vi "_readBoolean.vi"(8 "error in (no error)":errorcluster, 11 "tJSONParser in":refnum<class "tJSONParser.lvclass">) -> (0 "error out":errorcluster, 2 "tBSONBoolean out":refnum<class "tBSONBoolean.lvclass">, 3 "tJSONParser out":refnum<class "tJSONParser.lvclass">)   [LabVIEW 2013, in "JSON.lvlib" / "tJSONParser.lvclass"]
doc: "Reads and validates a boolean value from a string : value pair."
uses:
  tJSONParser.lvclass
  BSON/BSONElements/tBSONBoolean/tBSONBoolean.lvclass
  _error.ctl
  BSON/BSONElements/tBSONBoolean/setValue.vi
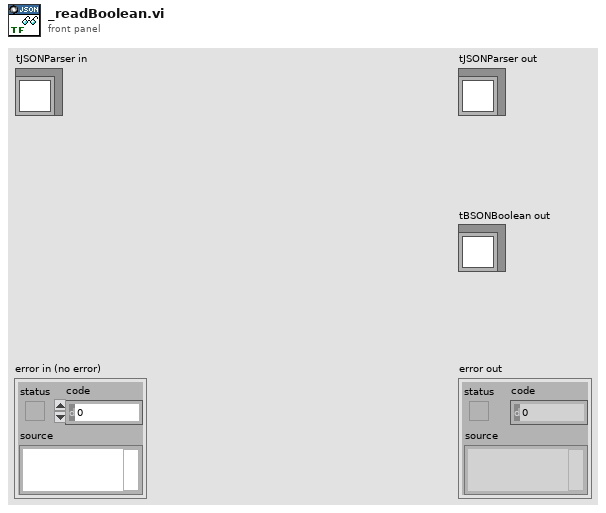
[diagram p1: front panel]
types:
  T1 = typedef "JSON.lvlib/tJSONParser.lvclass/_error.ctl" = enum16{"Missing Object Open", "Missing Pair Separator", "Missing Object End Or Separator", "Missing Pair String", "Unexpected Token", "Missing Array End Or Separator", "Invalid Escape Sequence", "Unexpected End Of File", "Invalid Unicode", "Unexpected End Of Line", "Invalid Numerical Constant"}
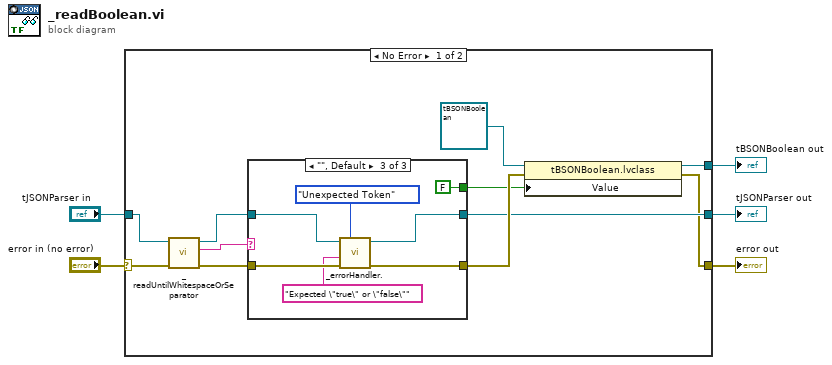
[diagram p0: block diagram]
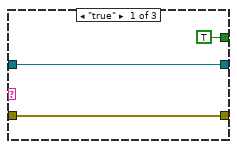
[diagram p2: hidden frame]
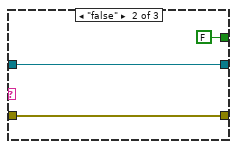
[diagram p3: hidden frame]
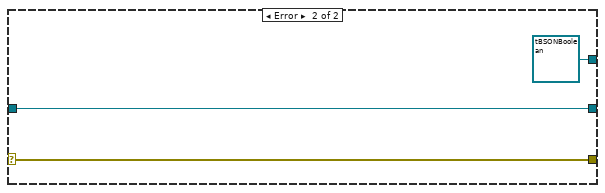
[diagram p4: hidden frame]
diagram:
  n1 = case shown="No Error" "error in (no error)" {
    selector: "error in (no error)" -> [w16 w32]
    tunnel: [w11 w32] -> w4
    tunnel: [w12 w31] -> w2
    tunnel: "tJSONParser in" -> [w8 w31]
    tunnel: [w10 refnum<class "tBSONBoolean.lvclass"> refnum ("lvMongoDriver.lvlib:BSON.lvlib:tBSONBoolean.lvclass")] -> w1
    frame No Error {
      n2 = call "_readUntilWhitespaceOrSeparator.vi"("error in (no error)"=w16, "tJSONParser in"=w8) -> ("error out"=w6:errorcluster, "String Out"=w7:string, "tJSONParser out"=w15:refnum<class "tJSONParser.lvclass">)  [unwired: 7 in]
      n3 = case shown="\"\", Default" w7 {
        tunnel: w6 -> [w18 w22 w29]
        tunnel: w15 -> [w19 w21 w28]
        tunnel: [w19 w21 w25] -> w12
        tunnel: [w18 w22 w24] -> w13
        tunnel: [TRUE FALSE FALSE] -> w9
        frame "true" {
        }
        frame "false" {
        }
        frame "", Default {
          n4 = call "_errorHandler..vi"("error in (no error)"=w29, "Additional Text"="Expected \"true\" or \"false\"", "Error Type"=_error."Unexpected Token", "JSON Parser In"=w28) -> ("error out"=w24:errorcluster, "JSON Parser Out"=w25:refnum<class "tJSONParser.lvclass">)  [unwired: 6 in]
        }
      }
      n5 = property class="tBSONBoolean.lvclass"(reference=refnum<class "tBSONBoolean.lvclass"> refnum ("lvMongoDriver.lvlib:BSON.lvlib:tBSONBoolean.lvclass"), error in=w13, "Value"=w9) -> (reference out=w10:refnum<class "tBSONBoolean.lvclass">, error out=w11:errorcluster)
    }
    frame Error {
    }
  }
  "error out" <- w4
  "tJSONParser out" <- w2
  "tBSONBoolean out" <- w1
